vi "QUERY_RECORD.vi"(8 "error in (no error)":errorcluster caption="错误输入（无错误）", 10 "sn":string="sn=") -> (0 "error out":errorcluster caption="错误输出", 1 "body":string, 2 "进站成功":bool)   [LabVIEW 2015]
uses:
  Global.vi
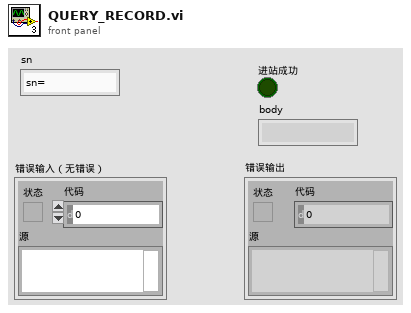
[diagram p1: front panel]
types:
  T1 = cluster{"URL":string, "audit_mode":string, "tsid":string, "model":string, "product":string, "test_station":string, "station_id":string, "test_station_name":string, "Webservice":string}
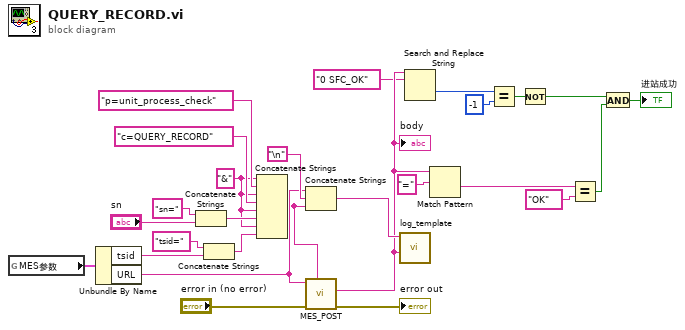
[diagram p0: block diagram]
diagram:
  w19 = "&"
  n1 = global read "Global.vi" "MES参数"() -> (w25:T1)
  n2 = Unbundle By Name(w25) -> ("tsid"=w14:string, "URL"=w13:string)
  n3 = Concatenate Strings("sn=", "sn") -> (w20:string)
  n4 = Concatenate Strings("tsid=", w14) -> (w18:string)
  n5 = Concatenate Strings(w19, "p=unit_process_check", w19, "c=QUERY_RECORD", w19, w20, w19, w18) -> (w12:string)
  n6 = Concatenate Strings(w13, "\n", w12) -> (w16:string)
  n7 = call "MES_POST.vi"("DATA"=w12, "错误输入（无错误）"="error in (no error)", "URL"=w13) -> ("错误输出"=→"error out":errorcluster, "body"=w6:string)  [unwired: 6 in, 1 out]
  "body" <- w6
  n8 = call "log_template.vi"("接收报文"=w6, "发送报文"=w16) -> ()  [unwired: 10 in]
  n9 = Search and Replace String(input string=w6, search string="0 SFC_OK") -> (offset past replacement=w4:i32)  [unwired: 6 in, 3 out]
  n10 = Match Pattern(string=w6, regular expression="=" ("正则表达式")) -> (after substring=w9:string)  [unwired: 1 in, 3 out]
  n11 = Equal?(x=w4, y=-1) -> (x = y?=w2:bool)
  n12 = Not(x=w2) -> (.not. x?=w1:bool)
  n13 = Equal?(x=w9, y="OK") -> (x = y?=w8:bool)
  n14 = And(x=w1, y=w8) -> (x .and. y?=→"进站成功":bool)
